vi "WaveformFGV.vi"(8 "error in":errorcluster, 10 "Set_Get":u16(ring) items=["Set", "Get"], 11 "Waveform":enum16{"Continous", "Ramped", "Pulsed"}(ring)) -> (0 "error out":errorcluster, 2 "Waveform":enum16{"Continous", "Ramped", "Pulsed"}(ring))   [LabVIEW 2010]
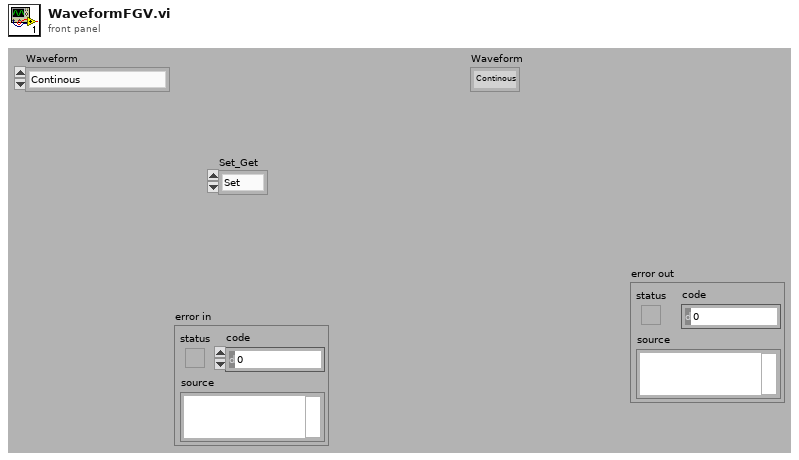
[diagram p1: front panel]
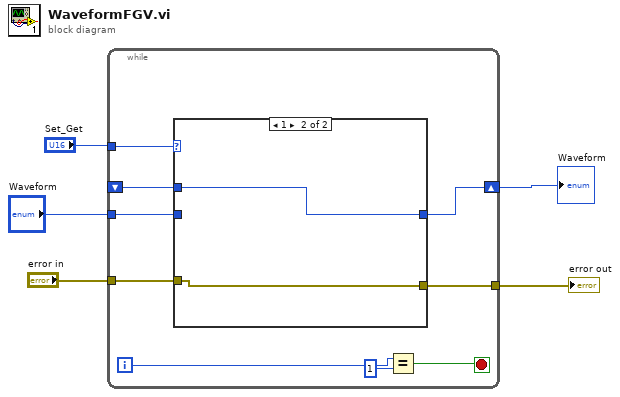
[diagram p0: block diagram]
diagram:
  n1 = while {
    tunnel: "Set_Get" -> [w14]
    tunnel: "Waveform" -> [w13]
    shift-right: [w12] -> w3
    shift-left: _ -> [w11]
    tunnel: [w7] -> w2
    tunnel: "error in" -> [w6]
    i -> [w9]
    stop <- w10 stop-if-true
    n2 = case shown="1" w14 {
      tunnel: w13 -> [w16 _]
      tunnel: [w16 w18] -> w12
      tunnel: w11 -> [_ w18]
      tunnel: [w15 w17] -> w7
      tunnel: w6 -> [w15 w17]
      frame 0, Default {
      }
      frame 1 {
      }
    }
    n3 = Equal?(x=w9, y=1) -> (x = y?=w10:bool)
  }
  "Waveform" <- w3
  "error out" <- w2
